vi "update values subvi.vi"(0 "UI Actor in":refnum<class "UI Actor.lvclass">, 1 "Message Enquuer":refnum<class "Message Enqueuer.lvclass">, 2 "Soda?":bool, 3 "Credito":dbl, 5 "MXN?":bool, 7 "Coins Enquuer":refnum<class "Message Enqueuer.lvclass">, 9 "Products Enquuer":refnum<class "Message Enqueuer.lvclass">, 12 "Producto":string, 13 "Costo":dbl, 14 "Inventario":dbl) -> (4 "UI Actor out":refnum<class "UI Actor.lvclass">)   [LabVIEW 2020, in "UI Actor.lvlib" / "UI Actor.lvclass"]
uses:
  UI Actor.lvclass
  <vilib>/ActorFramework/Message Enqueuer/Message Enqueuer.lvclass
  C:/Program Files (x86)/National Instruments/LabVIEW 2020/vi.lib/ActorFramework/Actor/Actor.lvclass
  UI Actor.lvclass/UI Actor.ctl
  <vilib>/ActorFramework/Actor/Actor.lvclass/Actor.ctl
  USD Actor Messages/Update Coins Msg/Update Coins Msg.lvclass/Update Coins Msg.ctl
  <vilib>/ActorFramework/Message Enqueuer/Message Enqueuer.lvclass/Message Enqueuer.ctl
  MXN Actor Messages/Update Coins Msg/Update Coins Msg.lvclass/Update Coins Msg.ctl
  UI Actor Messages/creditUpdate Msg/creditUpdate Msg.lvclass/creditUpdate Msg.ctl
  MSG Messages/Update MSG Msg/Update MSG Msg.lvclass/Update MSG Msg.ctl
  <vilib>/ActorFramework/Message Enqueuer/Enqueue.vi
  USD Actor Messages/Update Coins Msg/Update Coins Msg.lvclass
  C:/Program Files (x86)/National Instruments/LabVIEW 2020/vi.lib/ActorFramework/Message/Message.lvclass
  MXN Actor Messages/Update Coins Msg/Update Coins Msg.lvclass
  UI Actor Messages/creditUpdate Msg/creditUpdate Msg.lvclass
  MSG Messages/Update MSG Msg/Update MSG Msg.lvclass
  <vilib>/ActorFramework/Message Priority Queue/Priority Enqueue.vi
  <vilib>/ActorFramework/Actor/Actor.lvclass
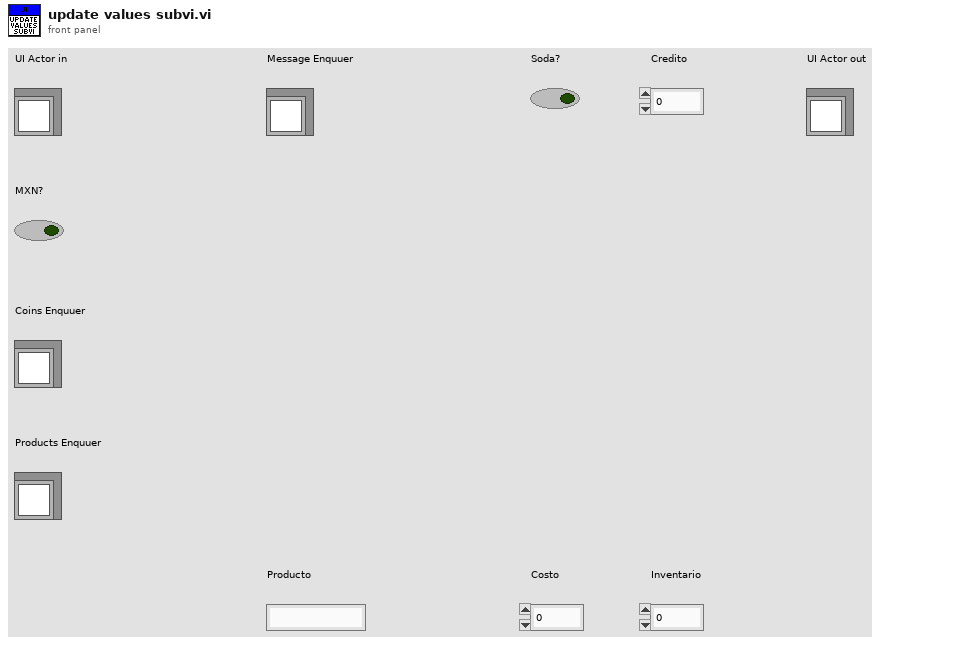
[diagram p1: front panel]
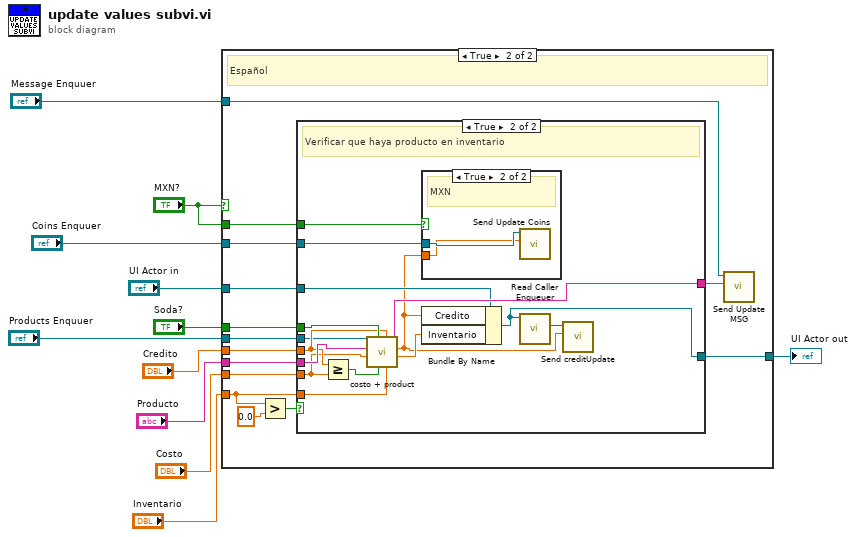
[diagram p0: block diagram]
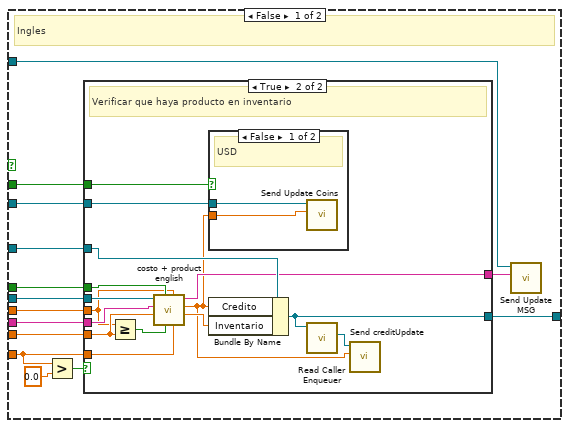
[diagram p2: hidden frame]
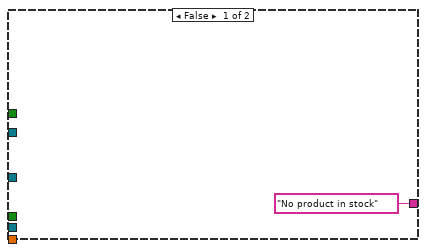
[diagram p3: hidden frame]
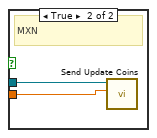
[diagram p4: hidden frame]
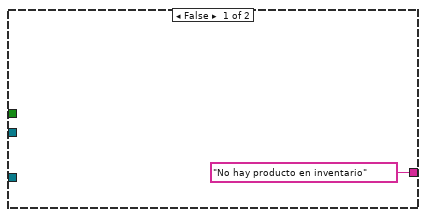
[diagram p5: hidden frame]
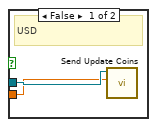
[diagram p6: hidden frame]
diagram:
  n1 = case shown="True" "MXN?" {
    tunnel: "Producto" -> [w17 w59]
    tunnel: "Soda?" -> [w18 w58]
    tunnel: "Credito" -> [w19 w57]
    tunnel: "Costo" -> [w16 w56]
    tunnel: "Message Enquuer" -> [w22 w54]
    tunnel: "UI Actor in" -> [w13 w51]
    tunnel: [w12 w50] -> w7
    tunnel: "Inventario" -> [w15 w49]
    tunnel: "Products Enquuer" -> [w20 w48]
    tunnel: "MXN?" -> [w14 w47]
    tunnel: "Coins Enquuer" -> [w21 w46]
    frame False {
      # "Ingles"
      n2 = Greater?(x=w15, y=0.0) -> (0:w24:bool)
      n3 = case shown="True" w24 {
        tunnel: w17 -> [_ w34]
        tunnel: w18 -> [_ w33]
        tunnel: w19 -> [_ w27]
        tunnel: w16 -> [_ w32]
        tunnel: ["No product in stock" w35] -> w25
        tunnel: w13 -> [_ w41]
        tunnel: [_ w40] -> w12
        tunnel: w15 -> [_ w30]
        tunnel: w20 -> [_ w36]
        tunnel: w14 -> [_ w38]
        tunnel: w21 -> [_ w37]
        frame False {
        }
        frame True {
          # "Verificar que haya producto en inventario"
          n4 = Greater Or Equal?(x=w27, y=w32) -> (x >= y?=w31:bool)
          n5 = call "costo + product english.vi"("Inventario"=w30, "Credito"=w27, "Boolean"=w31, "Soda?"=w33, "Costo"=w32, "Producto"=w34, "Message Enqueuer in"=w36) -> ("Numeric 2"=w29:dbl, "Numeric"=w28:dbl, "String"=w35:string)  [unwired: 2 in]
          n6 = case shown="False" w38 {
            tunnel: w37 -> [w43 w45]
            tunnel: w28 -> [w42 w44]
            frame False {
              # "USD"
              n7 = call "Send Update Coins.vi"("Credito Update"=w42, "Message Enqueuer"=w43) -> ()  [unwired: 8 in, 2 out]
            }
            frame True {
              # "MXN"
              n8 = call "Send Update Coins.vi"("Credito Update"=w44, "Message Enqueuer"=w45) -> ()  [unwired: 8 in, 2 out]
            }
          }
          n9 = Bundle By Name(cluster=w41, "Credito"=w28, "Inventario"=w29) -> (w40:refnum<class "UI Actor.lvclass">)
          n10 = call <vilib>:"Read Caller Enqueuer.vi"("Actor"=w40) -> ("Caller Enqueuer"=w39:refnum<class "Message Enqueuer.lvclass">)  [unwired: 10 in]
          n11 = call "Send creditUpdate.vi"("Credit"=w28, "Message Enqueuer"=w39) -> ()  [unwired: 8 in, 2 out]
        }
      }
      n12 = call "Send Update MSG.vi"("Update message"=w25, "Message Enqueuer"=w22) -> ()  [unwired: 8 in, 2 out]
    }
    frame True {
      # "Español"
      n13 = Greater?(x=w49, y=0.0) -> (0:w53:bool)
      n14 = case shown="True" w53 {
        tunnel: w59 -> [_ w75]
        tunnel: w58 -> [_ w74]
        tunnel: w57 -> [_ w72]
        tunnel: w56 -> [_ w71]
        tunnel: ["No hay producto en inventario" w70] -> w55
        tunnel: w51 -> [_ w69]
        tunnel: [_ w68] -> w50
        tunnel: w49 -> [_ w67]
        tunnel: w48 -> [_ w66]
        tunnel: w47 -> [_ w63]
        tunnel: w46 -> [_ w62]
        frame False {
        }
        frame True {
          # "Verificar que haya producto en inventario"
          n15 = Greater Or Equal?(x=w72, y=w71) -> (x >= y?=w73:bool)
          n16 = call "costo + product.vi"("Inventario"=w67, "Credito"=w72, "Boolean"=w73, "Soda?"=w74, "Costo"=w71, "Producto"=w75, "Message Enqueuer in"=w66) -> ("Numeric 2"=w65:dbl, "Numeric"=w61:dbl, "String"=w70:string)  [unwired: 2 in]
          n17 = case shown="True" w63 {
            tunnel: w62 -> [w77 w79]
            tunnel: w61 -> [w76 w78]
            frame False {
              # "USD"
              n18 = call "Send Update Coins.vi"("Credito Update"=w76, "Message Enqueuer"=w77) -> ()  [unwired: 8 in, 2 out]
            }
            frame True {
              # "MXN"
              n19 = call "Send Update Coins.vi"("Credito Update"=w78, "Message Enqueuer"=w79) -> ()  [unwired: 8 in, 2 out]
            }
          }
          n20 = Bundle By Name(cluster=w69, "Credito"=w61, "Inventario"=w65) -> (w68:refnum<class "UI Actor.lvclass">)
          n21 = call <vilib>:"Read Caller Enqueuer.vi"("Actor"=w68) -> ("Caller Enqueuer"=w64:refnum<class "Message Enqueuer.lvclass">)  [unwired: 10 in]
          n22 = call "Send creditUpdate.vi"("Credit"=w61, "Message Enqueuer"=w64) -> ()  [unwired: 8 in, 2 out]
        }
      }
      n23 = call "Send Update MSG.vi"("Update message"=w55, "Message Enqueuer"=w54) -> ()  [unwired: 8 in, 2 out]
    }
  }
  "UI Actor out" <- w7
